vi "tcp_server.vi"() -> ()   [LabVIEW 2019]
panel:
  out "error_out":errorcluster
  out "server_status":string
  out "server_step":i32
  out "value":dbl
  in  "stop":bool
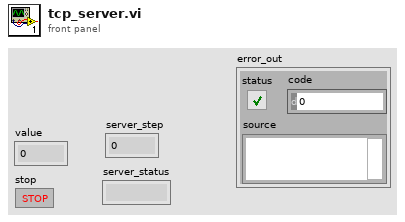
[diagram p1: front panel]
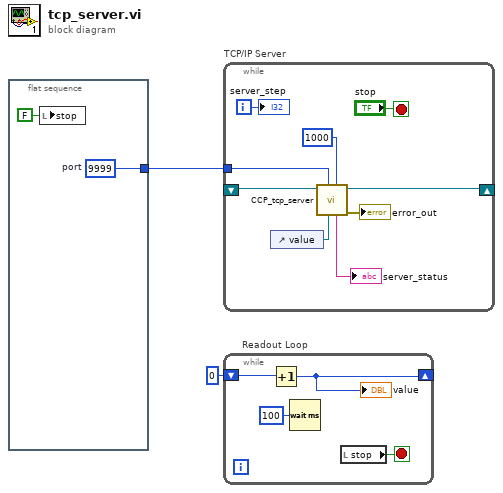
[diagram p0: block diagram]
diagram:
  n1 = flat-sequence {
    tunnel: [w3] -> w1
    frame #0 {
      w3 = u16 9999  # port
      n2 = local write "stop"(FALSE ("stop_server")) -> ()
    }
  }
  n3 = while "TCP/IP Server" {
    tunnel: w1 -> [w11]
    shift-right: [w6] -> _
    shift-left: _ -> [w7]
    i -> [w12]
    stop <- "stop" stop-if-true
    n4 = control-ref of="value"() -> (w8:refnum<vi>)
    n5 = call "CCP_tcp_server.vi"("timeout"=1000, "value"=w8, "port"=w11, "conn_id_in"=w7) -> ("error_out"=→"error_out":errorcluster, "conn_id_out"=w6:refnum<k5>, "status"=→"server_status":string)  [unwired: 5 in]
    "server_step" <- w12
  }
  n6 = while "Readout Loop" {
    shift-right: [w14] -> _
    shift-left: 0 -> [w17]
    stop <- w16 stop-if-true
    n7 = Increment(x=w17) -> (x+1=w14:i32)
    "value" <- w14
    n8 = Wait (ms)(milliseconds to wait=u32 100) -> ()  [unwired: 1 out]
    n9 = local read "stop"() -> (w16:bool)
  }
